vi "max_flow_correlation.vi"(1 "Current Flow Rate":dbl format="%#_13g", 2 "Current Voltage":dbl format="%#_13g") -> (0 "Max Flow Rate":dbl)   [LabVIEW 2015]
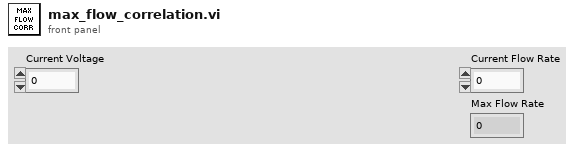
[diagram p1: front panel]
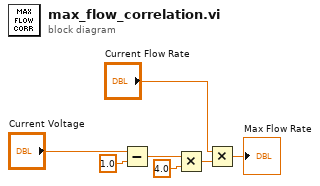
[diagram p0: block diagram]
diagram:
  n1 = Subtract(x="Current Voltage", y=1.0) -> (x-y=w5:dbl)
  n2 = Multiply(x=w5, y=4.0) -> (x*y=w3:dbl)
  n3 = Multiply(x="Current Flow Rate", y=w3) -> (x*y=→"Max Flow Rate":dbl)
